vi "HEWH RLT PRAT.vi"() -> ()   [LabVIEW 2023] (continued)
                      tunnel: w1999 -> [_ w2003]
                      frame False {
                      }
                      frame True {
                        n743 = Bundle By Name(cluster=w2005, "Station C Display.Display Data (RLT).Cycle Count Display"=w2003) -> (w2004:T97)
                      }
                    }
                  }
                  frame "D" {
                    n744 = case shown="False" w2009 {
                      tunnel: w2006 -> [w2010 w2013]
                      tunnel: [w2010 w2012] -> w2008
                      tunnel: w2007 -> [_ w2011]
                      frame False {
                      }
                      frame True {
                        n745 = Bundle By Name(cluster=w2013, "Station D Display.Display Data (RLT).Cycle Count Display"=w2011) -> (w2012:T97)
                      }
                    }
                  }
                }
              }
              event User Event {
                n746 = event-data() -> ()  [unwired: 1 in, 5 out]
                n747 = local read "Draw Station"() -> (w2017:string)
                n748 = case shown="\"A\"" w2017 {
                  tunnel: w2019 -> [w2025 w2029 w2036 w2042 w2050]
                  tunnel: [w2025 w2028 w2035 w2041 w2049] -> w2018
                  tunnel: w2016 -> [w2024 w2026 w2033 w2040 w2047]
                  tunnel: [w2024 w2026 w2033 w2040 w2047] -> w2015
                  frame Default {
                  }
                  frame "A" {
                    n749 = Unbundle By Name(w2029) -> ("Station A Display.Display Data (RLT)"=w2032:T32)
                    n750 = call "PRAT Update Status Color.vi"("Disable Cycle Counter"=FALSE, "Draw Station is Drawing Water"=TRUE, "Display Data (RLT) In"=w2032) -> ("Display Data (RLT) Out"=w2030:T32)  [unwired: 7 in, 1 out]
                    n751 = Bundle By Name(cluster=w2029, "Station A Display.Display Data (RLT)"=w2030) -> (w2028:T97)
                  }
                  frame "B" {
                    n752 = Unbundle By Name(w2036) -> ("Station B Display.Display Data (RLT)"=w2039:T32)
                    n753 = call "PRAT Update Status Color.vi"("Disable Cycle Counter"=FALSE, "Draw Station is Drawing Water"=TRUE, "Display Data (RLT) In"=w2039) -> ("Display Data (RLT) Out"=w2037:T32)  [unwired: 7 in, 1 out]
                    n754 = Bundle By Name(cluster=w2036, "Station B Display.Display Data (RLT)"=w2037) -> (w2035:T97)
                  }
                  frame "C" {
                    n755 = Unbundle By Name(w2042) -> ("Station C Display.Display Data (RLT)"=w2045:T32)
                    n756 = call "PRAT Update Status Color.vi"("Disable Cycle Counter"=FALSE, "Draw Station is Drawing Water"=TRUE, "Display Data (RLT) In"=w2045) -> ("Display Data (RLT) Out"=w2043:T32)  [unwired: 7 in, 1 out]
                    n757 = Bundle By Name(cluster=w2042, "Station C Display.Display Data (RLT)"=w2043) -> (w2041:T97)
                  }
                  frame "D" {
                    n758 = Unbundle By Name(w2050) -> ("Station D Display.Display Data (RLT)"=w2053:T32)
                    n759 = call "PRAT Update Status Color.vi"("Disable Cycle Counter"=FALSE, "Draw Station is Drawing Water"=TRUE, "Display Data (RLT) In"=w2053) -> ("Display Data (RLT) Out"=w2051:T32)  [unwired: 7 in, 1 out]
                    n760 = Bundle By Name(cluster=w2050, "Station D Display.Display Data (RLT)"=w2051) -> (w2049:T97)
                  }
                }
                n761 = flat-sequence {
                  tunnel: w2015 -> [w2022]
                  tunnel: [w2022] -> w2014
                  frame #0 {
                    n762 = local write "Start Draw"(FALSE ("Start Draw")) -> ()
                    n763 = local write "Draw Station"("") -> ()
                  }
                }
              }
              event "Start/Pause test": Value Change {
                n764 = event-data() -> ("NewVal"=w2059:bool)  [unwired: 1 in, 5 out]
                n765 = case shown="False" w2059 {
                  tunnel: w2060 -> [w2066 w2074]
                  tunnel: [w2064 w2074] -> w2058
                  tunnel: w2057 -> [w2062 w2073]
                  tunnel: [w2061 w2073] -> w2056
                  frame False {
                    n766 = global read "Save File Globals HCC.vi" "Startup"() -> (w2065:u32)
                    n767 = Bundle By Name(cluster=w2066, "Station A Display.Display Data (RLT).Status Color"=w2065, "Station B Display.Display Data (RLT).Status Color"=w2065, "Station C Display.Display Data (RLT).Status Color"=w2065, "Station D Display.Display Data (RLT).Status Color"=w2065) -> (w2064:T97)
                    n768 = for {
                      N: 10 -> [_]
                      shift-right: [w2068] -> w2061
                      shift-left: w2062 -> [w2069]
                      n769 = call "UTILITY Boolean Notifier.vi"("Status"=UTILITY_Notifier."Set", "error in (no error)"=w2069, "Set Status"=TRUE, "name (unnamed)"="Stop Custom Draw") -> ("error out"=w2068:errorcluster)  [unwired: 6 in, 1 out]
                      n770 = Wait Until Next ms Multiple(millisecond multiple=u32 10) -> ()  [unwired: 1 out]
                    }
                  }
                  frame True {
                  }
                }
                n771 = call <vilib>:"Add State(s) to Queue__jki_lib_state_machine.vi"("State(s) in (\"\")"=w2055) -> ("States Out"=w2054:string)  [unwired: 14 in]
              }
            }
          }
          frame "---------- Core ----------" {
            n772 = call <vilib>:"Add State(s) to Queue__jki_lib_state_machine.vi"("State(s) in (\"\")"=w2079) -> ("States Out"=w2078:string)  [unwired: 14 in]
          }
          frame Default {
            w2090 = 42 items=["No error", "Argument error", "Memory is full", "Out of zone", "End of file", "File already open", "Generic file I/O error", "File not found", "File permission error", "Disk is full", "Duplicate path", "Too many files open", "System feature not enabled", "Resource file not found", "Cannot add resource", "Resource not found", "Image not found", "Image memory error", "Pen does not exist", "Config type invalid", "Config token not found", "Config parse error", "Config memory error", "Bad external code format", "Bad external code offset", "External code not present", "Null window", "Destroy window error", "Null menu", "Print aborted", "Bad print record", "Print driver error", "Windows error during printing", "Memory error during printing", "Print dialog error", "Generic print error", "Invalid device refnum", "Device not found", "Device parameter error", "Device unit error", "Cannot open device", "Device call aborted", "Generic error", "Cancelled by user", "Object ID too low", "Object ID too high", "Object not in heap", "Unknown heap", "Unknown object (invalid DefProc)", "Unknown object (DefProc not in table)", "Message out of range", "Invalid (null) method", "Unknown message", "Manager call not supported", "Bad address", "Network operation in progress", "Network operation timed out", "Connection is busy", "Network attribute not supported", "Network error", "Address in use", "System out of memory", "Connection aborted", "Connection refused", "Not connected", "Already connected", "Connection closed", "Initialization error (interapplication manager)", "Bad occurrence", "Wait on unbound occurrence handler", "Occurrence queue overflow", "Datalog type conflict", "Unused", "Unrecognized type (interapplication manager)", "Memory corrupt", "Failed to make temporary DLL", "Old CIN version", "Drag socket not found", "Failed to load drop-object", "Failed to register OLE object", "Failed to release OLE object", "Format specifier type mismatch", "Unknown format specifier", "Too few format specifiers", "Too many format specifiers", "Scan failed", "Newer CIN version", "Error converting to variant", "Runtime menu error", "Password tampered", "Variant attribute not found", "Incompatible variant data type", "Event data is not available", "Event Store is not present", "Occurrence is not found", "Event Queue is not created", "Event info is not available", "Refnum passed is NULL", "Error retrieving Class GUID", "Error retrieving CoClass GUID", "Error retrieving TypeLib GUID.", "Bad built application magic bytes.", "Specific driver is different from the specific driver associated with the Logical Name.", "There is no session opened to the class driver.", "Max Error", "MAX - Error with config objects", "MAX - Error loading configuration", "MAX - Group not supported"]
            # "Current State"
            # "Handle mistyped state name (developer tool)"
            n773 = Format Into String(format string="Software Exception: Unhandled State \"%s\"." ("message"), error in=w2086, w2081) -> (resulting string=w2089:string, error out=w2088:errorcluster)  [unwired: 1 in]
            n774 = call <vilib>:"Error Cluster From Error Code.vi"("show call chain? (False)"=TRUE, "error in (no error)"=w2088, "error message (\"\")"=w2089, "error code (0)"=w2090) -> ("error out"=w2087:errorcluster)  [unwired: 5 in]
            n775 = call <vilib>:"Add State(s) to Queue__jki_lib_state_machine.vi"("State(s) in (\"\")"=w2085) -> ("States Out"=w2084:string)  [unwired: 14 in]
          }
          frame "Initialize Core Data" {
            # "If panel starts closed or is an EXE, then close it when we exit"
            n776 = property class="App"() -> ("App.Kind"=w2099:T94)  [unwired: 2 in, 2 out]
            n777 = control-ref of="Current VI Reference"() -> (w2093:refnum<vi>)
            n778 = property class="VI"() -> ("Front Panel.Open"=w2100:bool)  [unwired: 2 in, 2 out]
            n779 = Not(x=w2100) -> (.not. x?=w2097:bool)
            n780 = Equal?(x=w2099, y=T94."Run Time System" ("Application:Kind")) -> (x = y?=w2096:bool)
            n781 = Or(x=w2097, y=w2096) -> (x .or. y?=w2094:bool)
            n782 = Bundle By Name(cluster=w2095, "Core.Current VI Reference"=w2093, "Core.Close Panel on Exit?"=w2094) -> (w2102:T97)
            n783 = call <vilib>:"Add State(s) to Queue__jki_lib_state_machine.vi"("State(s) in (\"\")"=w2104) -> ("States Out"=w2103:string)  [unwired: 14 in]
          }
          frame "Initialize Channels" {
            n784 = disable-structure shown="Enabled" {
              disable-tunnel: w2109 -> [w2140 _]
              disable-tunnel: w2108 -> [w2136 w2141]
              disable-tunnel: [w2131 w2141] -> w2107
              disable-tunnel: [w2117 _] -> w2105
              frame Disabled {
                w2127 = T98 0 items=["both", "start of string", "end of string"] ("location (both)")
                # "The channel list is compiled here"
                n785 = local read "LV Program"() -> (w2118:T25)
                n786 = call "HEWH RLT Channel Test Labels.vi"("LV Program"=w2118, "Error In"=w2136) -> ("Station A"=w2135:T99, "Station B"=w2134:T99, "Station C"=w2133:T99, "Station D"=w2132:T99, "Error Out"=w2131:errorcluster)  [unwired: 9 in]
                n787 = call "HEWH RLT Label Parse.vi"("Station A"=w2135) -> ("Agilent Channel List"=w2122:string[][], "MW100 Channel List"=w2123:string[][])  [unwired: 6 in, 3 out]
                n788 = call "HEWH RLT Label Parse.vi"("Station A"=w2134) -> ("Agilent Channel List"=w2120:string[][], "MW100 Channel List"=w2121:string[][])  [unwired: 6 in, 3 out]
                n789 = call "HEWH RLT Label Parse.vi"("Station A"=w2133) -> ("Agilent Channel List"=w2125:string[][], "MW100 Channel List"=w2126:string[][])  [unwired: 6 in, 3 out]
                n790 = call "HEWH RLT Label Parse.vi"("Station A"=w2132) -> ("Agilent Channel List"=w2124:string[][], "MW100 Channel List"=w2119:string[][])  [unwired: 6 in, 3 out]
                n791 = Build Array (concatenate)(w2122, w2120, w2125, w2124) -> (w2129:string[][])
                n792 = Index Array(array=w2129, index (col)=1 ("disabled index (col)")) -> (element=w2128:string[])  [unwired: 1 in]
                n793 = Array To Spreadsheet String(delimiter (Tab)="," ("format string"), array=w2128, 3:"%s" ("format string")) -> (spreadsheet string=w2137:string)
                n794 = call <vilib>:"Trim Whitespace.vi"("string"=w2137, "location (both)"=w2127) -> ("trimmed string"=w2115:string)
                "Analog Channel-List" <- w2115
                n795 = Bundle By Name(cluster=w2140, "RLT Station Channels.MW100.Station A Channels, MW100"=w2123, "RLT Station Channels.Agilent.Station A Channels, Agilent"=w2122, "RLT Station Channels.MW100.Station B Channels, MW100"=w2121, "RLT Station Channels.Agilent.Station B Channels, Agilent"=w2120, "RLT Station Channels.Agilent.Station C Channels, Agilent"=w2125, "RLT Station Channels.MW100.Station C Channels, MW100"=w2126, "RLT Station Channels.Agilent.Station D Channels, Agilent"=w2124, "RLT Station Channels.MW100.Station D Channels, MW100"=w2119) -> (w2117:T97)
                n796 = Equal?(x=w2115, y="") -> (x = y?=w2113:bool)
                n797 = Not(x=w2113) -> (.not. x?=→"Use Agilent?":bool)
                n798 = Unbundle By Name(w2117) -> ("RLT Station Channels"=w2116:T54)
                n799 = local write "RLT Station Channels"(w2116) -> ()
              }
              frame Enabled {
              }
            }
            n800 = call <vilib>:"Add State(s) to Queue__jki_lib_state_machine.vi"("State(s) in (\"\")"=w2111) -> ("States Out"=w2110:string)  [unwired: 14 in]
          }
          frame "Initialize Files" {
            n801 = Bundle By Name(cluster=w2148, "Station A Display"=w2145, "Station B Display"=w2144, "Station C Display"=w2143, "Station D Display"=w2142) -> (w2147:T97)
            n802 = call <vilib>:"Add State(s) to Queue__jki_lib_state_machine.vi"("State(s) in (\"\")"=w2151) -> ("States Out"=w2150:string)  [unwired: 14 in]
          }
          frame "Init Complete" {
            n803 = Unbundle By Name(w2168) -> ("Station A Display.Display Data (RLT)"=w2169:T32, "Station B Display.Display Data (RLT)"=w2162:T32, "Station C Display.Display Data (RLT)"=w2161:T32, "Station D Display.Display Data (RLT)"=w2160:T32)
            n804 = call "PRAT Update Status Color.vi"("Disable Cycle Counter"=TRUE, "Disable Station"=HEWH_RLT_Station_Disable."Disable Station (No Draw)", "Display Data (RLT) In"=w2169) -> ("Display Data (RLT) Out"=w2158:T32)  [unwired: 7 in, 1 out]
            n805 = call "PRAT Update Status Color.vi"("Disable Cycle Counter"=TRUE, "Disable Station"=HEWH_RLT_Station_Disable."Disable Station (No Draw)", "Display Data (RLT) In"=w2162) -> ("Display Data (RLT) Out"=w2157:T32)  [unwired: 7 in, 1 out]
            n806 = call "PRAT Update Status Color.vi"("Disable Cycle Counter"=TRUE, "Disable Station"=HEWH_RLT_Station_Disable."Disable Station (No Draw)", "Display Data (RLT) In"=w2161) -> ("Display Data (RLT) Out"=w2156:T32)  [unwired: 7 in, 1 out]
            n807 = call "PRAT Update Status Color.vi"("Disable Cycle Counter"=TRUE, "Disable Station"=HEWH_RLT_Station_Disable."Disable Station (No Draw)", "Display Data (RLT) In"=w2160) -> ("Display Data (RLT) Out"=w2155:T32)  [unwired: 7 in, 1 out]
            n808 = call <vilib>:"Add State(s) to Queue__jki_lib_state_machine.vi"("State(s) in (\"\")"=w2182) -> ("States Out"=w2181:string)  [unwired: 14 in]
            n809 = call "UTILITY String Notifier.vi"("Status"=UTILITY_Notifier."Set", "error in (no error)"=w2170, "Set Status"="", "name (unnamed)"="Draw Station") -> ("error out"=w2172:errorcluster)  [unwired: 6 in, 1 out]
            n810 = Bundle By Name(cluster=w2168, "Station A Display.Display Data (RLT)"=w2158, "Station B Display.Display Data (RLT)"=w2157, "Station C Display.Display Data (RLT)"=w2156, "Station D Display.Display Data (RLT)"=w2155) -> (w2167:T97)
            n811 = call "UTILITY String Notifier.vi"("Status"=UTILITY_Notifier."Set", "error in (no error)"=w2172, "Set Status"=T8 "Initializing Complete...." ("Message"), "name (unnamed)"="Message") -> ("error out"=w2173:errorcluster)  [unwired: 6 in, 1 out]
            "Init Complete" <- TRUE ("Init Complete")
          }
          frame "Save Status" {
            n812 = Unbundle By Name(w2201) -> ("Station A Display"=w2199:T31, "Station B Display"=w2196:T31, "Station C Display"=w2186:T31, "Station D Display"=w2185:T31)
            n813 = local read "File Locations A"() -> (w2198:T3)
            n814 = call "HCC Read Write Display.vi"("Read Write Control"=enum16{"Read", "Write"}."Write", "error in (no error)"=w2184, "Washer Input"=w2199, "File Locations In"=w2198) -> ("error out"=w2193:errorcluster)  [unwired: 6 in, 1 out]
            n815 = local read "File Locations B"() -> (w2195:T3)
            n816 = call "HCC Read Write Display.vi"("Read Write Control"=enum16{"Read", "Write"}."Write", "error in (no error)"=w2193, "Washer Input"=w2196, "File Locations In"=w2195) -> ("error out"=w2190:errorcluster)  [unwired: 6 in, 1 out]
            n817 = local read "File Locations C"() -> (w2192:T3)
            n818 = call "HCC Read Write Display.vi"("Read Write Control"=enum16{"Read", "Write"}."Write", "error in (no error)"=w2190, "Washer Input"=w2186, "File Locations In"=w2192) -> ("error out"=w2187:errorcluster)  [unwired: 6 in, 1 out]
            n819 = local read "File Locations D"() -> (w2189:T3)
            n820 = call "HCC Read Write Display.vi"("Read Write Control"=enum16{"Read", "Write"}."Write", "error in (no error)"=w2187, "Washer Input"=w2185, "File Locations In"=w2189) -> ("error out"=w2183:errorcluster)  [unwired: 6 in, 1 out]
            n821 = call <vilib>:"Add State(s) to Queue__jki_lib_state_machine.vi"("State(s) in (\"\")"=w2203) -> ("States Out"=w2202:string)  [unwired: 14 in]
          }
          frame "Error Handler" {
            # "Unhandled Error -- Display it"
            n822 = call <vilib>:"General Error Handler.vi"("error in (no error)"=w2205) -> ()  [unwired: 10 in, 5 out]
            n823 = call <vilib>:"Add State(s) to Queue__jki_lib_state_machine.vi"("State(s) in Front (\"\")"="/* Post Error States", "State(s) in (\"\")"=w2207) -> ("States Out"=w2210:string)  [unwired: 13 in]
          }
          frame "Exit" {
            n824 = call <vilib>:"Add State(s) to Queue__jki_lib_state_machine.vi"("State(s) in (\"\")"=w2216) -> ("States Out"=w2215:string)  [unwired: 14 in]
          }
          frame "---------- Data ----------" {
            n825 = call <vilib>:"Add State(s) to Queue__jki_lib_state_machine.vi"("State(s) in (\"\")"=w2221) -> ("States Out"=w2220:string)  [unwired: 14 in]
          }
          frame "Data: Initialize" {
            n826 = flat-sequence {
              tunnel: [w2237] -> w2223
              frame #0 {
              }
              frame #1 {
                w2228 = HEWH_Special_Condition_Check."N/A"  # Current Cond D
                w2229 = HEWH_Special_Condition_Check."N/A"  # Current Cond C
                w2230 = HEWH_Special_Condition_Check."N/A"  # Current Cond B
                w2231 = HEWH_Special_Condition_Check."N/A"  # Current Cond A
                w2239 = errorcluster[] []  # Error Log
                w2240 = i32[] []  # DrawsLeft
                n827 = local read "Power Analyzer"() -> (w2227:T12)
                n828 = Bundle("Core"=T95 {"Current VI Reference"=refnum, "Close Panel on Exit?"=FALSE}, "DrawsLeft"=w2240, "Error Log"=w2239, "RLT Station Channels"="RLT Station Channels", "Station A Display"="Station A Display", "Station B Display"="Station B Display", "Station C Display"="Station C Display", "Station D Display"="Station D Display", "Draw Parameters Seq"=T48 {"Draws Left"=0, "Draws Left Array"=[], "Remaining Draws (A)"=1000, "Remaining Draws (B)"=1000, "Remaining Draws (C)"=1000, "Remaining Draws (D)"=1000, "Index of Element (A-D)"=[], "Station A"={"Sequence #"=0.0, "Cycles"=0, "Mode Setting"="", "Flow Rate (GPM)"=0.0, "Temperature (F)"=0.0, "Reset Timer"=FALSE, "Use Temp Decline Method"=FALSE, "Terminate Condition"=enum."C1-Terminate Draw @ Gallon Mark", "Condition Value #1"=0.0, "UE"=FALSE, "LE"=FALSE, "Comp"=FALSE, "Fan"=FALSE, "Test End Time (Sec)"=0.0, "Purge Until Cutout"=FALSE, "Start Conditions"=enum."Heat Source Cutout", "Condition Value #2"=0.0, "Remove Power"=FALSE, "Time"=0.0, "Check Special Cond."=enum."SC2-Check Heat Source (On-C2/Off-C1)", "Condition#"=enum."C1", "Draw Flags"=enum."N/A", "Data Processing Delay (FHD 15sec, UEF 5 Sec)"=0.0, "Test Complete"=FALSE, "User Setpoint"=0.0, "Tank Setpoint"=0.0}, "Station B"={"Sequence #"=0.0, "Cycles"=0, "Mode Setting"="", "Flow Rate (GPM)"=0.0, "Temperature (F)"=0.0, "Reset Timer"=FALSE, "Use Temp Decline Method"=FALSE, "Terminate Condition"=enum."C1-Terminate Draw @ Gallon Mark", "Condition Value #1"=0.0, "UE"=FALSE, "LE"=FALSE, "Comp"=FALSE, "Fan"=FALSE, "Test End Time (Sec)"=0.0, "Purge Until Cutout"=FALSE, "Start Conditions"=enum."Heat Source Cutout", "Condition Value #2"=0.0, "Remove Power"=FALSE, "Time"=0.0, "Check Special Cond."=enum."SC2-Check Heat Source (On-C2/Off-C1)", "Condition#"=enum."C1", "Draw Flags"=enum."N/A", "Data Processing Delay (FHD 15sec, UEF 5 Sec)"=0.0, "Test Complete"=FALSE, "User Setpoint"=0.0, "Tank Setpoint"=0.0}, "Station C"={"Sequence #"=0.0, "Cycles"=0, "Mode Setting"="", "Flow Rate (GPM)"=0.0, "Temperature (F)"=0.0, "Reset Timer"=FALSE, "Use Temp Decline Method"=FALSE, "Terminate Condition"=enum."C1-Terminate Draw @ Gallon Mark", "Condition Value #1"=0.0, "UE"=FALSE, "LE"=FALSE, "Comp"=FALSE, "Fan"=FALSE, "Test End Time (Sec)"=0.0, "Purge Until Cutout"=FALSE, "Start Conditions"=enum."Heat Source Cutout", "Condition Value #2"=0.0, "Remove Power"=FALSE, "Time"=0.0, "Check Special Cond."=enum."SC2-Check Heat Source (On-C2/Off-C1)", "Condition#"=enum."C1", "Draw Flags"=enum."N/A", "Data Processing Delay (FHD 15sec, UEF 5 Sec)"=0.0, "Test Complete"=FALSE, "User Setpoint"=0.0, "Tank Setpoint"=0.0}, "Station D"={"Sequence #"=0.0, "Cycles"=0, "Mode Setting"="", "Flow Rate (GPM)"=0.0, "Temperature (F)"=0.0, "Reset Timer"=FALSE, "Use Temp Decline Method"=FALSE, "Terminate Condition"=enum."C1-Terminate Draw @ Gallon Mark", "Condition Value #1"=0.0, "UE"=FALSE, "LE"=FALSE, "Comp"=FALSE, "Fan"=FALSE, "Test End Time (Sec)"=0.0, "Purge Until Cutout"=FALSE, "Start Conditions"=enum."Heat Source Cutout", "Condition Value #2"=0.0, "Remove Power"=FALSE, "Time"=0.0, "Check Special Cond."=enum."SC2-Check Heat Source (On-C2/Off-C1)", "Condition#"=enum."C1", "Draw Flags"=enum."N/A", "Data Processing Delay (FHD 15sec, UEF 5 Sec)"=0.0, "Test Complete"=FALSE, "User Setpoint"=0.0, "Tank Setpoint"=0.0}}, "Current Cond A"=w2231, "Current Cond B"=w2230, "Current Cond C"=w2229, "Current Cond D"=w2228, "Power Analyzer"=w2227) -> (w2237:T97)  [unwired: 1 in]
              }
            }
            n829 = call <vilib>:"Add State(s) to Queue__jki_lib_state_machine.vi"("State(s) in (\"\")"=w2226) -> ("States Out"=w2225:string)  [unwired: 14 in]
          }
          frame "Data: Cleanup" {
            n830 = Unbundle By Name(w2246) -> ("Core.Current VI Reference"=w2245:refnum<vi>)
            n831 = Close Reference(reference=w2245, error in (no error)=w2244) -> (error out=w2242:errorcluster)
            n832 = call <vilib>:"Add State(s) to Queue__jki_lib_state_machine.vi"("State(s) in (\"\")"=w2248) -> ("States Out"=w2247:string)  [unwired: 14 in]
          }
          frame "---------- UI ----------" {
            n833 = call <vilib>:"Add State(s) to Queue__jki_lib_state_machine.vi"("State(s) in (\"\")"=w2253) -> ("States Out"=w2252:string)  [unwired: 14 in]
          }
          frame "UI: Initialize" {
            n834 = local read "LV Program"() -> (w2254:T25)
            n835 = local write "Init Complete"(FALSE ("Recording Data")) -> ()
            n836 = case shown="Default" w2254 {
              tunnel: w2254 -> [w2262 _ _]
              frame Default {
                w2264 = T87."Disabled and Grayed Out" ("Disabled")
                w2265 = HEWH_RLT_Station_Disable."Disable Station (No Draw)" ("Disable Station 2")
                w2266 = T87."Disabled and Grayed Out" ("Disabled")
                w2269 = FALSE ("DAQ for B")
                w2270 = T87."Disabled and Grayed Out" ("Disabled")
                n837 = flat-sequence {
                  tunnel: w2262 -> [w2288]
                  frame #0 {
                    w2275 = T87."Disabled and Grayed Out" ("Disabled")
                    w2277 = T87."Disabled and Grayed Out" ("Disabled")
                    w2282 = T87."Disabled and Grayed Out" ("Disabled")
                    w2287 = T87."Enabled" ("Disabled")
                    n838 = property on="Inlet Valve A" class="CmbBox (strict)"("DisabledEnum"=T87."Enabled" ("Disabled")) -> (error out=w2283:errorcluster)  [unwired: 2 in, 1 out]
                    n839 = property on="Drain Valve A" class="CmbBox (strict)"("DisabledEnum"=T87."Enabled" ("Disabled")) -> (error out=w2280:errorcluster)  [unwired: 2 in, 1 out]
                    n840 = property on="Outlet Valve A" class="CmbBox (strict)"("DisabledEnum"=T87."Enabled" ("Disabled")) -> (error out=w2274:errorcluster)  [unwired: 2 in, 1 out]
                    n841 = property on="IF Start" class="Bool"("DisabledEnum"=w2287) -> ()  [unwired: 2 in, 2 out]
                    n842 = property on="Inlet Valve B" class="CmbBox (strict)"(error in=w2283, "DisabledEnum"=w2282) -> (error out=w2285:errorcluster)  [unwired: 1 in, 1 out]
                    n843 = property on="Drain Valve B" class="CmbBox (strict)"(error in=w2280, "DisabledEnum"=w2277) -> (error out=w2279:errorcluster)  [unwired: 1 in, 1 out]
                    n844 = property on="Outlet Valve B" class="CmbBox (strict)"(error in=w2274, "DisabledEnum"=w2275) -> (error out=w2273:errorcluster)  [unwired: 1 in, 1 out]
                    n845 = property on="IF Stop" class="Bool"("DisabledEnum"=w2287) -> ()  [unwired: 2 in, 2 out]
                    n846 = property on="Inlet Valve C" class="CmbBox (strict)"(error in=w2285, "DisabledEnum"=w2282) -> (error out=w2284:errorcluster)  [unwired: 1 in, 1 out]
                    n847 = property on="Drain Valve C" class="CmbBox (strict)"(error in=w2279, "DisabledEnum"=w2277) -> (error out=w2278:errorcluster)  [unwired: 1 in, 1 out]
                    n848 = property on="Outlet Valve C" class="CmbBox (strict)"(error in=w2273, "DisabledEnum"=w2275) -> (error out=w2272:errorcluster)  [unwired: 1 in, 1 out]
                    n849 = property on="Main Power" class="Bool (strict)"("DisabledEnum"=w2287) -> ()  [unwired: 2 in, 2 out]
                    n850 = property on="Inlet Valve D" class="CmbBox (strict)"(error in=w2284, "DisabledEnum"=w2282) -> ()  [unwired: 1 in, 2 out]
                    n851 = property on="Drain Valve D" class="CmbBox (strict)"(error in=w2278, "DisabledEnum"=w2277) -> ()  [unwired: 1 in, 2 out]
                    n852 = property on="Outlet Valve D" class="CmbBox (strict)"(error in=w2272, "DisabledEnum"=w2275) -> ()  [unwired: 1 in, 2 out]
                  }
                  frame #1 {
                    n853 = case shown="\"Gas Water Heater\"" w2288 {
                      frame Default {
                        w2289 = FALSE ("Get Gas Data")
                        w2290 = T87."Disabled and Grayed Out" ("Disabled")
                        n854 = property on="Start ANSI UI" class="Bool (strict)"("DisabledEnum"=w2290) -> ()  [unwired: 2 in, 2 out]
                        n855 = property on="Tare Meter" class="Bool"("DisabledEnum"=w2290) -> ()  [unwired: 2 in, 2 out]
                        n856 = property on="Reset Totalizer" class="Bool"("DisabledEnum"=w2290) -> ()  [unwired: 2 in, 2 out]
                      }
                      frame "Gas Water Heater" {
                        w2291 = TRUE ("Get Gas Data")
                        w2292 = T87."Enabled" ("Disabled")
                        n857 = property on="Start ANSI UI" class="Bool (strict)"("DisabledEnum"=w2292) -> ()  [unwired: 2 in, 2 out]
                        n858 = property on="Tare Meter" class="Bool"("DisabledEnum"=w2292) -> ()  [unwired: 2 in, 2 out]
                        n859 = property on="Reset Totalizer" class="Bool"("DisabledEnum"=w2292) -> ()  [unwired: 2 in, 2 out]
                      }
                    }
                  }
                }
                n860 = property on="Trigger Draw B" class="Bool"("DisabledEnum"=w2264) -> ()  [unwired: 2 in, 2 out]
                n861 = property on="Trigger Draw C" class="Bool"("DisabledEnum"=w2264) -> ()  [unwired: 2 in, 2 out]
                n862 = property on="Trigger Draw D" class="Bool"("DisabledEnum"=w2264) -> ()  [unwired: 2 in, 2 out]
                n863 = property on="DAQ for A" class="Bool (strict)"("DisabledEnum"=T87."Enabled" ("Disabled")) -> ()  [unwired: 2 in, 2 out]
                n864 = property on="DAQ for B" class="Bool (strict)"("DisabledEnum"=w2270) -> ()  [unwired: 2 in, 2 out]
                n865 = property on="DAQ for C" class="Bool (strict)"("DisabledEnum"=w2270) -> ()  [unwired: 2 in, 2 out]
                n866 = property on="DAQ for D" class="Bool (strict)"("DisabledEnum"=w2270) -> ()  [unwired: 2 in, 2 out]
                n867 = local write "DAQ for B"(w2269) -> ()
                n868 = local write "DAQ for D"(w2269) -> ()
                n869 = local write "DAQ for A"(TRUE ("DAQ for A")) -> ()
                n870 = local write "DAQ for C"(w2269) -> ()
                n871 = property on="Disable Station 1" class="Enum (strict)"("DisabledEnum"=T87."Enabled" ("Disabled")) -> ()  [unwired: 2 in, 2 out]
                n872 = property on="Disable Station 2" class="Enum (strict)"("DisabledEnum"=w2266) -> ()  [unwired: 2 in, 2 out]
                n873 = property on="Disable Station 3" class="Enum (strict)"("DisabledEnum"=w2266) -> ()  [unwired: 2 in, 2 out]
                n874 = property on="Disable Station 4" class="Enum (strict)"("DisabledEnum"=w2266) -> ()  [unwired: 2 in, 2 out]
                n875 = property on="Disable Station 2" class="Enum (strict)"("Value"=w2265) -> ()  [unwired: 2 in, 2 out]
                n876 = property on="Disable Station 3" class="Enum (strict)"("Value"=w2265) -> ()  [unwired: 2 in, 2 out]
                n877 = property on="Disable Station 4" class="Enum (strict)"("Value"=w2265) -> ()  [unwired: 2 in, 2 out]
                n878 = property on="Trigger Draw A" class="Bool"("DisabledEnum"=T87."Enabled" ("Disabled")) -> ()  [unwired: 2 in, 2 out]
              }
              frame "HEWH RLT" {
                w2293 = FALSE ("DAQ for B")
                w2297 = T87."Enabled" ("Disabled")
                w2299 = T87."Enabled" ("Disabled")
                w2304 = T87."Enabled" ("Disabled")
                w2309 = T87."Enabled" ("Disabled")
                w2310 = T87."Enabled" ("Disabled")
                w2312 = T87."Enabled" ("Disabled")
                w2311 = T87."Enabled" ("Disabled")
                n879 = property on="Disable Station 1" class="Enum (strict)"("DisabledEnum"=w2310) -> ()  [unwired: 2 in, 2 out]
                n880 = property on="Trigger Draw A" class="Bool"("DisabledEnum"=w2309) -> ()  [unwired: 2 in, 2 out]
                n881 = property on="DAQ for A" class="Bool (strict)"("DisabledEnum"=w2312) -> ()  [unwired: 2 in, 2 out]
                n882 = property on="Drain Valve A" class="CmbBox (strict)"("DisabledEnum"=T87."Enabled" ("Disabled")) -> (error out=w2302:errorcluster)  [unwired: 2 in, 1 out]
                n883 = property on="Outlet Valve A" class="CmbBox (strict)"("DisabledEnum"=T87."Enabled" ("Disabled")) -> (error out=w2296:errorcluster)  [unwired: 2 in, 1 out]
                n884 = property on="Inlet Valve A" class="CmbBox (strict)"("DisabledEnum"=T87."Enabled" ("Disabled")) -> (error out=w2305:errorcluster)  [unwired: 2 in, 1 out]
                n885 = property on="IF Start" class="Bool"("DisabledEnum"=w2311) -> ()  [unwired: 2 in, 2 out]
                n886 = property on="DAQ for B" class="Bool (strict)"("DisabledEnum"=w2312) -> ()  [unwired: 2 in, 2 out]
                n887 = property on="IF Stop" class="Bool"("DisabledEnum"=w2311) -> ()  [unwired: 2 in, 2 out]
                n888 = property on="Drain Valve B" class="CmbBox (strict)"(error in=w2302, "DisabledEnum"=w2299) -> (error out=w2301:errorcluster)  [unwired: 1 in, 1 out]
                n889 = property on="Outlet Valve B" class="CmbBox (strict)"(error in=w2296, "DisabledEnum"=w2297) -> (error out=w2295:errorcluster)  [unwired: 1 in, 1 out]
                n890 = property on="Inlet Valve B" class="CmbBox (strict)"(error in=w2305, "DisabledEnum"=w2304) -> (error out=w2307:errorcluster)  [unwired: 1 in, 1 out]
                n891 = property on="Trigger Draw B" class="Bool"("DisabledEnum"=w2309) -> ()  [unwired: 2 in, 2 out]
                n892 = property on="Disable Station 2" class="Enum (strict)"("DisabledEnum"=w2310) -> ()  [unwired: 2 in, 2 out]
                n893 = property on="DAQ for C" class="Bool (strict)"("DisabledEnum"=w2312) -> ()  [unwired: 2 in, 2 out]
                n894 = property on="Main Power" class="Bool (strict)"("DisabledEnum"=w2311) -> ()  [unwired: 2 in, 2 out]
                n895 = property on="Drain Valve C" class="CmbBox (strict)"(error in=w2301, "DisabledEnum"=w2299) -> (error out=w2300:errorcluster)  [unwired: 1 in, 1 out]
                n896 = property on="Outlet Valve C" class="CmbBox (strict)"(error in=w2295, "DisabledEnum"=w2297) -> (error out=w2294:errorcluster)  [unwired: 1 in, 1 out]
                n897 = property on="Inlet Valve C" class="CmbBox (strict)"(error in=w2307, "DisabledEnum"=w2304) -> (error out=w2306:errorcluster)  [unwired: 1 in, 1 out]
                n898 = property on="Trigger Draw C" class="Bool"("DisabledEnum"=w2309) -> ()  [unwired: 2 in, 2 out]
                n899 = property on="DAQ for D" class="Bool (strict)"("DisabledEnum"=w2312) -> ()  [unwired: 2 in, 2 out]
                n900 = property on="Disable Station 3" class="Enum (strict)"("DisabledEnum"=w2310) -> ()  [unwired: 2 in, 2 out]
                n901 = property on="Drain Valve D" class="CmbBox (strict)"(error in=w2300, "DisabledEnum"=w2299) -> ()  [unwired: 1 in, 2 out]
                n902 = property on="Outlet Valve D" class="CmbBox (strict)"(error in=w2294, "DisabledEnum"=w2297) -> ()  [unwired: 1 in, 2 out]
                n903 = property on="Inlet Valve D" class="CmbBox (strict)"(error in=w2306, "DisabledEnum"=w2304) -> ()  [unwired: 1 in, 2 out]
                n904 = property on="Trigger Draw D" class="Bool"("DisabledEnum"=w2309) -> ()  [unwired: 2 in, 2 out]
                n905 = property on="Disable Station 4" class="Enum (strict)"("DisabledEnum"=w2310) -> ()  [unwired: 2 in, 2 out]
                n906 = local write "DAQ for B"(w2293) -> ()
                n907 = local write "DAQ for D"(w2293) -> ()
                n908 = local write "DAQ for C"(w2293) -> ()
                n909 = local write "DAQ for A"(w2293) -> ()
              }
              frame "PRAT" {
                w2313 = FALSE ("DAQ for B")
                w2317 = T87."Disabled and Grayed Out" ("Disabled")
                w2319 = T87."Disabled and Grayed Out" ("Disabled")
                w2324 = T87."Enabled" ("Disabled")
                w2329 = T87."Enabled" ("Disabled")
                w2330 = T87."Enabled" ("Disabled")
                w2332 = T87."Disabled and Grayed Out" ("Disabled")
                w2331 = T87."Disabled and Grayed Out" ("Disabled")
                n910 = property on="DAQ for A" class="Bool (strict)"("DisabledEnum"=w2332) -> ()  [unwired: 2 in, 2 out]
                n911 = property on="Outlet Valve A" class="CmbBox (strict)"("DisabledEnum"=T87."Disabled and Grayed Out" ("Disabled")) -> (error out=w2316:errorcluster)  [unwired: 2 in, 1 out]
                n912 = property on="Disable Station 1" class="Enum (strict)"("DisabledEnum"=w2330) -> ()  [unwired: 2 in, 2 out]
                n913 = property on="Trigger Draw A" class="Bool"("DisabledEnum"=w2329) -> ()  [unwired: 2 in, 2 out]
                n914 = property on="Drain Valve A" class="CmbBox (strict)"("DisabledEnum"=T87."Disabled and Grayed Out" ("Disabled")) -> (error out=w2322:errorcluster)  [unwired: 2 in, 1 out]
                n915 = property on="Inlet Valve A" class="CmbBox (strict)"("DisabledEnum"=T87."Enabled" ("Disabled")) -> (error out=w2325:errorcluster)  [unwired: 2 in, 1 out]
                n916 = property on="IF Start" class="Bool"("DisabledEnum"=w2331) -> ()  [unwired: 2 in, 2 out]
                n917 = property on="DAQ for B" class="Bool (strict)"("DisabledEnum"=w2332) -> ()  [unwired: 2 in, 2 out]
                n918 = property on="IF Stop" class="Bool"("DisabledEnum"=w2331) -> ()  [unwired: 2 in, 2 out]
                n919 = property on="Outlet Valve B" class="CmbBox (strict)"(error in=w2316, "DisabledEnum"=w2317) -> (error out=w2315:errorcluster)  [unwired: 1 in, 1 out]
                n920 = property on="Drain Valve B" class="CmbBox (strict)"(error in=w2322, "DisabledEnum"=w2319) -> (error out=w2321:errorcluster)  [unwired: 1 in, 1 out]
                n921 = property on="Inlet Valve B" class="CmbBox (strict)"(error in=w2325, "DisabledEnum"=w2324) -> (error out=w2327:errorcluster)  [unwired: 1 in, 1 out]
                n922 = property on="Trigger Draw B" class="Bool"("DisabledEnum"=w2329) -> ()  [unwired: 2 in, 2 out]
                n923 = property on="Disable Station 2" class="Enum (strict)"("DisabledEnum"=w2330) -> ()  [unwired: 2 in, 2 out]
                n924 = property on="DAQ for C" class="Bool (strict)"("DisabledEnum"=w2332) -> ()  [unwired: 2 in, 2 out]
                n925 = property on="Main Power" class="Bool (strict)"("DisabledEnum"=w2331) -> ()  [unwired: 2 in, 2 out]
                n926 = property on="Outlet Valve C" class="CmbBox (strict)"(error in=w2315, "DisabledEnum"=w2317) -> (error out=w2314:errorcluster)  [unwired: 1 in, 1 out]
                n927 = property on="Drain Valve C" class="CmbBox (strict)"(error in=w2321, "DisabledEnum"=w2319) -> (error out=w2320:errorcluster)  [unwired: 1 in, 1 out]
                n928 = property on="Inlet Valve C" class="CmbBox (strict)"(error in=w2327, "DisabledEnum"=w2324) -> (error out=w2326:errorcluster)  [unwired: 1 in, 1 out]
                n929 = property on="Trigger Draw C" class="Bool"("DisabledEnum"=w2329) -> ()  [unwired: 2 in, 2 out]
                n930 = property on="DAQ for D" class="Bool (strict)"("DisabledEnum"=w2332) -> ()  [unwired: 2 in, 2 out]
                n931 = property on="Disable Station 3" class="Enum (strict)"("DisabledEnum"=w2330) -> ()  [unwired: 2 in, 2 out]
                n932 = property on="Outlet Valve D" class="CmbBox (strict)"(error in=w2314, "DisabledEnum"=w2317) -> ()  [unwired: 1 in, 2 out]
                n933 = property on="Drain Valve D" class="CmbBox (strict)"(error in=w2320, "DisabledEnum"=w2319) -> ()  [unwired: 1 in, 2 out]
                n934 = property on="Inlet Valve D" class="CmbBox (strict)"(error in=w2326, "DisabledEnum"=w2324) -> ()  [unwired: 1 in, 2 out]
                n935 = property on="Trigger Draw D" class="Bool"("DisabledEnum"=w2329) -> ()  [unwired: 2 in, 2 out]
                n936 = property on="Disable Station 4" class="Enum (strict)"("DisabledEnum"=w2330) -> ()  [unwired: 2 in, 2 out]
                n937 = local write "DAQ for B"(w2313) -> ()
                n938 = local write "DAQ for D"(w2313) -> ()
                n939 = local write "DAQ for C"(w2313) -> ()
                n940 = local write "DAQ for A"(w2313) -> ()
              }
            }
            n941 = call <vilib>:"Add State(s) to Queue__jki_lib_state_machine.vi"("State(s) in (\"\")"=w2261) -> ("States Out"=w2260:string)  [unwired: 14 in]
            n942 = property on="Start/Pause test" class="Bool (strict)"("DisabledEnum"=T87."Disabled and Grayed Out" ("Disabled")) -> ()  [unwired: 2 in, 2 out]
          }
          frame "UI: Cursor Set" {
            # "Argument"
            # "Set and Unset Cursor Busy.\n(Usage: \"UI: Cursor Set >> Busy|Idle\")"
            n943 = case shown="\"Busy\"" w2334 {
              tunnel: w2336 -> [w2341 w2343]
              tunnel: [w2340 w2342] -> w2335
              frame "Idle", Default {
                n944 = call <vilib>:"Unset Busy.vi"("error in (no error)"=w2341) -> ("error out"=w2340:errorcluster)  [unwired: 10 in]
              }
              frame "Busy" {
                n945 = call <vilib>:"Set Busy.vi"("error in (no error)"=w2343) -> ("error out"=w2342:errorcluster)  [unwired: 9 in, 1 out]
              }
            }
            n946 = call <vilib>:"Add State(s) to Queue__jki_lib_state_machine.vi"("State(s) in (\"\")"=w2339) -> ("States Out"=w2338:string)  [unwired: 14 in]
          }
          frame "UI: Front Panel State" {
            # "Argument"
            n947 = Unbundle By Name(w2347) -> ("Core.Current VI Reference"=w2346:refnum<vi>)
            n948 = case shown="\"Open\", Default" w2345 {
              tunnel: w2349 -> [w2355 w2368]
              tunnel: [w2357 w2369] -> w2348
              tunnel: w2346 -> [w2356 w2366]
              frame "Open", Default {
                n949 = property class="VI"(reference=w2356, error in=w2355) -> (reference out=w2353:refnum<vi>, error out=w2354:errorcluster, "Front Panel.Open"=w2352:bool)
                n950 = case shown="False" w2352 {
                  tunnel: [w2360 w2363] -> w2357
                  tunnel: w2354 -> [w2359 w2363]
                  tunnel: w2353 -> [w2358 _]
                  frame False {
                    n951 = invoke class="VI" method="FP.Open"(reference=w2358, error in=w2359, "Activate"=TRUE, "State"=T96."Maximized") -> (error out=w2360:errorcluster)  [unwired: 1 in, 4 out]
                  }
                  frame True {
                  }
                }
              }
              frame "Close" {
                n952 = property class="VI"(reference=w2366, error in=w2368) -> (reference out=w2365:refnum<vi>, error out=w2367:errorcluster, "Front Panel.Open"=w2364:bool)
                n953 = case shown="False" w2364 {
                  tunnel: [w2370 w2373] -> w2369
                  tunnel: w2367 -> [w2370 w2372]
                  tunnel: w2365 -> [_ w2371]
                  frame False {
                  }
                  frame True {
                    n954 = disable-structure shown="Enabled" {
                      disable-tunnel: [w2376 w2377] -> w2373
                      disable-tunnel: w2372 -> [w2375 w2377]
                      disable-tunnel: w2371 -> [w2374 _]
                      frame Disabled {
                        n955 = invoke class="VI" method="FP.Close"(reference=w2374, error in=w2375) -> (error out=w2376:errorcluster)  [unwired: 1 in, 2 out]
                      }
                      frame Enabled {
                      }
                    }
                  }
                }
              }
            }
            n956 = call <vilib>:"Add State(s) to Queue__jki_lib_state_machine.vi"("State(s) in (\"\")"=w2351) -> ("States Out"=w2350:string)  [unwired: 14 in]
          }
          frame "---------- Macro ----------" {
            n957 = call <vilib>:"Add State(s) to Queue__jki_lib_state_machine.vi"("State(s) in (\"\")"=w2382) -> ("States Out"=w2381:string)  [unwired: 14 in]
          }
          frame "Macro: Initialize" {
            w2384 = "Data: Initialize\nInitialize Core Data\nUI: Initialize\nUI: Front Panel State >> Open\nInitialize Channels\nInitialize Files\nTest: Update Display A\nTest: Update Display B\nTest: Update Display C\nTest: Update Display D\nInit Complete"  # Data: Initialize Initialize Core Data UI: Initialize UI: Front Panel State >> Open Initialize Channels Initialize Files Test: Update Display A Test: Update Display B Test: Update Display C Test: Update Display D Init Complete
            n958 = call <vilib>:"Add State(s) to Queue__jki_lib_state_machine.vi"("State(s) in Front (\"\")"=w2384, "State(s) in (\"\")"=w2388) -> ("States Out"=w2387:string)  [unwired: 13 in]
          }
          frame "Macro: Exit" {
            n959 = Unbundle By Name(w2396) -> ("Core.Close Panel on Exit?"=w2395:bool)
            n960 = Select(t="UI: Front Panel State >> Close", s=w2395, f="") -> (s? t:f=w2392:string)
            n961 = call <vilib>:"Add State(s) to Queue__jki_lib_state_machine.vi"("State(s) in (\"\")"=w2392, "State(s) at Back (\"\")"="Data: Cleanup\nExit") -> ("States Out"=w2390:string)  [unwired: 13 in]
            n962 = call <vilib>:"Add State(s) to Queue__jki_lib_state_machine.vi"("State(s) in Front (\"\")"=w2390, "State(s) in (\"\")"=w2399) -> ("States Out"=w2398:string)  [unwired: 13 in]
          }
          frame "---------- Test ----------" {
            n963 = call <vilib>:"Add State(s) to Queue__jki_lib_state_machine.vi"("State(s) in (\"\")"=w2404) -> ("States Out"=w2403:string)  [unwired: 14 in]
          }
          frame "Test: Check Complete" {
            n964 = local read "Station D Test Sequence"() -> (w2430:T15[])
            n965 = local read "Use Last Start Condition B?"() -> (w2419:bool)
            n966 = local read "Use Last Start Condition D?"() -> (w2417:bool)
            n967 = local read "Station A Test Sequence"() -> (w2433:T15[])
            n968 = local read "Station B Test Sequence"() -> (w2432:T15[])
            n969 = local read "Station C Test Sequence"() -> (w2431:T15[])
            n970 = local read "Use Last Start Condition A?"() -> (w2420:bool)
            n971 = local read "Use Last Start Condition C?"() -> (w2418:bool)
            n972 = Unbundle By Name(w2434) -> ("Station A Display.Display Data (RLT).Cycle Count Display"=w2426:i32, "Station A Display.Display Data (RLT).Cycle Count Display"=w2427:i32, "Station A Display.Display Data (RLT).Cycle Count Display"=w2428:i32, "Station A Display.Display Data (RLT).Cycle Count Display"=w2429:i32)
            n973 = call "PRAT Multi Station Check.vi"("Station A Test Sequence"=w2433, "Station B Test Sequence"=w2432, "Station C Test Sequence"=w2431, "Station D Test Sequence"=w2430, "Error In"=w2425, "Cycle Count Display (Station A)"=w2429, "Use Last Start Condition A?"=w2420, "Cycle Count Display (Station B)"=w2428, "Cycle Count Display (Station C)"=w2427, "Use Last Start Condition B?"=w2419, "Cycle Count Display (Station D)"=w2426, "Use Last Start Condition C?"=w2418, "Use Last Start Condition D?"=w2417) -> ("Draw Parameters"=w2416:T48, "Error Out"=w2407:errorcluster)  [unwired: 13 in]
            "Current Draw Parameters" <- w2416
            n974 = Unbundle By Name(w2416) -> ("Remaining Draws (A)"=→"Remaining Draws (A)":i32, "Remaining Draws (B)"=→"Remaining Draws (B)":i32, "Remaining Draws (C)"=→"Remaining Draws (C)":i32, "Remaining Draws (D)"=→"Remaining Draws (D)":i32, "Draws Left"=w2415:i32)
            "Draws Left" <- w2415
            n975 = local read "Log Data Output (D)"() -> (w2412:bool)
            n976 = local read "Log Data Output (C)"() -> (w2411:bool)
            n977 = local read "LV Program"() -> (w2408:T25)
            n978 = local read "Log Data Output (A)"() -> (w2414:bool)
            n979 = local read "Log Data Output (B)"() -> (w2413:bool)
            n980 = call "HEWH Create Save Data States.vi"("LV Program"=w2408, "Data Loop?"=FALSE, "Error In"=w2407, "Log Data Output (C)"=w2411, "Log Data Output (A)"=w2414, "Log Data Output (D)"=w2412, "Log Data Output (B)"=w2413) -> ("SM States"=w2409:string, "Error Out"=w2406:errorcluster)  [unwired: 11 in]
            n981 = case shown="0" w2415 {
              tunnel: w2406 -> [w2440 w2444]
              tunnel: [w2439 w2444] -> w2405
              frame 0 {
                n982 = call "UTILITY String Notifier.vi"("Status"=UTILITY_Notifier."Set", "error in (no error)"=w2440, "Set Status"=T8 "All Draws Complete..." ("Message"), "name (unnamed)"="Message") -> ("error out"=w2439:errorcluster)  [unwired: 6 in, 1 out]
              }
              frame 1, Default {
              }
            }
            n983 = Bundle By Name(cluster=w2434, "Draw Parameters Seq"=w2416) -> (w2436:T97)
            n984 = call <vilib>:"Add State(s) to Queue__jki_lib_state_machine.vi"("State(s) in Front (\"\")"=w2409, "State(s) in (\"\")"=w2438) -> ("States Out"=w2437:string)  [unwired: 13 in]
          }
          frame "Test: Update Display A" {
            n985 = local read "Appliance Details A"() -> (w2445:T5)
            n986 = local read "Current (A)"() -> (w2454:dbl)
            n987 = Bundle By Name(cluster=w2455, "Station A Display.Display Data (RLT).Current Display"=w2454, "Station A Display.Appliance Details"=w2445) -> (w2453:T97)
            n988 = Unbundle By Name(w2453) -> ("Station A Display.Display Data (RLT).Station Label Display"=w2451:string, "Station A Display.Display Data (RLT).Board ID Display"=w2450:string, "Station A Display.Display Data (RLT).Serial Number Display"=w2449:string, "Station A Display.Display Data (RLT).Current Display"=w2448:dbl, "Station A Display.Display Data (RLT).Status Color"=w2447:u32, "Station A Display.Display Data (RLT).Cycle Count Display"=w2446:i32)
            n989 = property on="Station Label Display" class="Str"("Value"=w2451) -> ()  [unwired: 2 in, 2 out]
            n990 = property on="Board ID Display" class="Str"("Value"=w2450) -> ()  [unwired: 2 in, 2 out]
            n991 = property on="Serial Number Display" class="Str"("Value"=w2449) -> ()  [unwired: 2 in, 2 out]
            n992 = property on="Current Display" class="DigNum (strict)"("Value"=w2448) -> ()  [unwired: 2 in, 2 out]
            n993 = property on="Status Color" class="ColBox"("Value"=w2447) -> ()  [unwired: 2 in, 2 out]
            n994 = property on="Cycle Count Display" class="DigNum (strict)"("Value"=w2446) -> ()  [unwired: 2 in, 2 out]
            n995 = call <vilib>:"Add State(s) to Queue__jki_lib_state_machine.vi"("State(s) in (\"\")"=w2458) -> ("States Out"=w2457:string)  [unwired: 14 in]
          }
          frame "Test: Update Display B" {
            n996 = local read "Appliance Details B"() -> (w2459:T5)
            n997 = local read "Current (B)"() -> (w2468:dbl)
            n998 = Bundle By Name(cluster=w2469, "Station B Display.Display Data (RLT).Current Display"=w2468, "Station B Display.Appliance Details"=w2459) -> (w2467:T97)
            n999 = Unbundle By Name(w2467) -> ("Station B Display.Display Data (RLT).Station Label Display"=w2465:string, "Station B Display.Display Data (RLT).Board ID Display"=w2464:string, "Station B Display.Display Data (RLT).Serial Number Display"=w2463:string, "Station B Display.Display Data (RLT).Current Display"=w2462:dbl, "Station B Display.Display Data (RLT).Status Color"=w2461:u32, "Station B Display.Display Data (RLT).Cycle Count Display"=w2460:i32)
            n1000 = property on="Cycle Count Display" class="DigNum (strict)"("Value"=w2460) -> ()  [unwired: 2 in, 2 out]
            n1001 = property on="Current Display" class="DigNum (strict)"("Value"=w2462) -> ()  [unwired: 2 in, 2 out]
            n1002 = property on="Station Label Display" class="Str"("Value"=w2465) -> ()  [unwired: 2 in, 2 out]
            n1003 = property on="Board ID Display" class="Str"("Value"=w2464) -> ()  [unwired: 2 in, 2 out]
            n1004 = property on="Serial Number Display" class="Str"("Value"=w2463) -> ()  [unwired: 2 in, 2 out]
            n1005 = property on="Status Color" class="ColBox"("Value"=w2461) -> ()  [unwired: 2 in, 2 out]
